vi "UTIL_Get Project Directory v1_0_0.vi"(8 "error in (no error)":errorcluster, 11 "path":path) -> (0 "error out":errorcluster, 3 "project directory":path)   [LabVIEW 2015]
doc: "UTIL_Get Project Directory.vi\n\nReturns the current project directory Or working path of the calling VI\n\nCreated 2006 by \n\nJ. Daren Suntych\nNational Analytics\n970-397-0764"
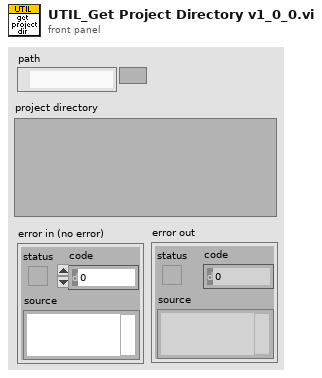
[diagram p1: front panel]
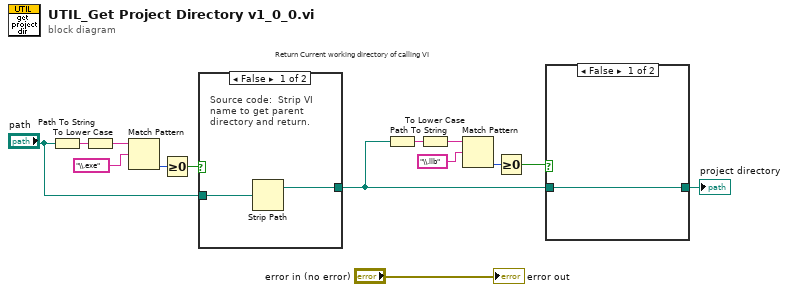
[diagram p0: block diagram]
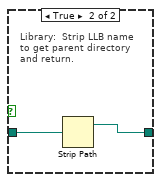
[diagram p2: hidden frame]
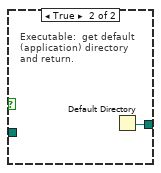
[diagram p3: hidden frame]
diagram:
  # "Return Current working directory of calling VI"
  n1 = Path To String(path="path") -> (string=w14:string)
  n2 = To Lower Case(string=w14) -> (all lower case string=w12:string)
  n3 = Match Pattern(string=w12, regular expression="\\.exe") -> (offset past match=w11:i32)  [unwired: 4 out]
  n4 = Greater Or Equal To 0?(x=w11) -> (x >= 0?=w10:bool)
  n5 = case shown="False" w10 {
    tunnel: "path" -> [w16 _]
    tunnel: [w15 w17] -> w2
    frame False {
      # "Source code:  Strip VI name to get parent directory and return."
      n6 = Strip Path(path=w16) -> (stripped path=w15:path)  [unwired: 1 out]
    }
    frame True {
      # "Executable:  get default (application) directory and return."
      n7 = Default Directory() -> (w17:path)
    }
  }
  n8 = Path To String(path=w2) -> (string=w6:string)
  n9 = To Lower Case(string=w6) -> (all lower case string=w8:string)
  n10 = Match Pattern(string=w8, regular expression="\\.llb") -> (offset past match=w9:i32)  [unwired: 4 out]
  n11 = Greater Or Equal To 0?(x=w9) -> (x >= 0?=w5:bool)
  n12 = case shown="False" w5 {
    tunnel: w2 -> [w18 w20]
    tunnel: [w18 w19] -> w1
    frame False {
    }
    frame True {
      # "Library:  Strip LLB name to get parent directory and return."
      n13 = Strip Path(path=w20) -> (stripped path=w19:path)  [unwired: 1 out]
    }
  }
  "project directory" <- w1
  "error out" <- "error in (no error)"
